vi "PH_gentec_Powermeter.Action get Info.vi"(0 "VI in":refnum<vi>, 5 "error in (no error)":errorcluster) -> (14 "VI out":refnum<vi>, 19 "error out":errorcluster)   [LabVIEW 2014, in "PH_gentec_Powermeter.lvlib"]
uses:
  PH_gentec_Powermeter.lvlib
  PH_Basics/PH_Powermeter_BaseClass/PH_Powermeter_BaseClass.State.ctl
  PH_Basics/PH_Powermeter_BaseClass/PH_Powermeter_BaseClass.lvlib
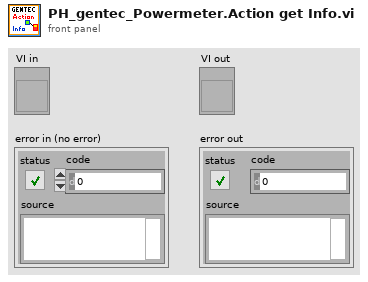
[diagram p1: front panel]
types:
  T1 = typedef "PH_Powermeter_BaseClass.lvlib/PH_Powermeter_BaseClass.State.ctl" = enum32{"off", "operating", "opened", "checked", "connected", "Sets to change", "running"}
  T2 = typedef "PH_Powermeter_BaseClass.lvlib/PH_Powermeter_BaseClass.i attribute.ctl" = cluster{"GUI References":T3, "Connection":T4, "Head Attributes":T5, "VISA resource":refnum<visa-resource-name>, "Energy":T6, "Service ID Energy":i32, "Wanted Settings":T7, "Current Settings":T7}
  T3 = typedef "PH_Powermeter_BaseClass.lvlib/PH_Powermeter_BaseClass.GUI Refs.ctl" = cluster{"Head Attributes":refnum<vi>, "Energy":refnum<vi>, "Connection":refnum<vi>, "VISA Resource":refnum<vi>, "Scaling Factor":refnum<vi>, "Range":refnum<vi>, "Wavelength":refnum<vi>, "Trigger Level":refnum<vi>, "Wanted Settings":refnum<vi>, "Current Settings":refnum<vi>}
  T4 = typedef "PH_Powermeter_BaseClass.lvlib/PH_Powermeter_BaseClass.Connection.ctl" = cluster{"failed checks":i8, "Timeout":bool, "Data read":string, "Failure":bool, "Error":bool, "State":T1}
  T5 = typedef "PH_Powermeter_BaseClass.lvlib/PH_Powermeter_BaseClass.Head Attributes.ctl" = cluster{"Instrument Type":string, "Head Version":string, "Head Name":string, "Serial Number":string, "Firmware":string, "Sensor Type":string, "MinimumRange":u32, "Maximum Range":u32, "Min Wavelength":i32, "Max Wavelength":i32}
  T6 = typedef "PH_Powermeter_BaseClass.lvlib/PH_Powermeter_BaseClass.Energy.ctl" = cluster{"current Value":dbl, "unscaled":dbl, "Scaling Factor":dbl}
  T7 = typedef "PH_Powermeter_BaseClass.lvlib/PH_gentec_BaseClass.Head Settings.ctl" = cluster{"Trigger Level":dbl, "Wavelength":u32, "Range":u32}
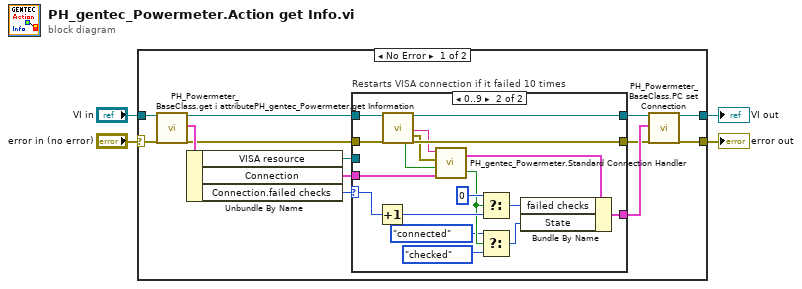
[diagram p0: block diagram]
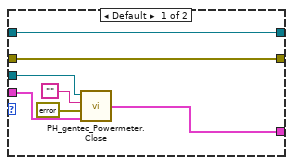
[diagram p2: hidden frame]
diagram:
  n1 = case shown="No Error" "error in (no error)" {
    selector: "error in (no error)" -> [w6 w43]
    tunnel: [w17 w43] -> w4
    tunnel: [w16 w44] -> w3
    tunnel: "VI in" -> [w7 w44]
    frame No Error {
      n2 = call "PH_Powermeter_BaseClass.get i attribute.vi"("i ref in"=w7, "error in (no error)"=w6) -> ("i ref out"=w8:refnum<vi>, "i attribute"=w11:T2, "error out"=w10:errorcluster)  [unwired: 15 in]
      n3 = Unbundle By Name(w11) -> ("VISA resource"=w5:refnum<visa-resource-name>, "Connection"=w12:T4, "Connection.failed checks"=w13:i8)
      n4 = case "Restarts VISA connection if it failed 10 times" shown="0..9" w13 {
        selector: w13 -> [_ w42]
        tunnel: w8 -> [w24 w41]
        tunnel: [w24 w40] -> w14
        tunnel: w10 -> [w23 w39]
        tunnel: [w23 w38] -> w9
        tunnel: w12 -> [w22 w37]
        tunnel: [w19 w32] -> w15
        tunnel: w5 -> [w18 _]
        frame Default {
          n5 = call "PH_gentec_Powermeter.Close.vi"("Connection in"=w22, "Device Error in"=errorcluster {"status"=FALSE, "code"=0, "source"=""} ("Device Error out"), "Error Message"="", "VISA Refnum in"=w18) -> ("Connection out"=w19:T4)
        }
        frame 0..9 {
          n6 = Increment(x=w42) -> (x+1=w30:i8)
          n7 = call "PH_gentec_Powermeter.get Information.vi"("i ref in"=w41, "error in"=w39) -> ("Timeout?"=w34:bool, "i ref out"=w40:refnum<vi>, "Error Messages"=w35:string, "Device Error out"=w36:errorcluster, "error out"=w38:errorcluster)  [unwired: 13 in]
          n8 = call "PH_gentec_Powermeter.Standard Connection Handler.vi"("Connection in"=w37, "Timeout"=w34, "Device Error"=w36, "Error"=w35) -> ("No problem"=w28:bool, "Connection out"=w33:T4)
          n9 = Select(t=i8 0, s=w28, f=w30) -> (s? t:f=w29:i8)
          n10 = Select(t=PH_Powermeter_BaseClass.State."connected" ("State"), s=w28, f=PH_Powermeter_BaseClass.State."checked") -> (s? t:f=w25:T1)
          n11 = Bundle By Name(cluster=w33, "failed checks"=w29, "State"=w25) -> (w32:T4)
        }
      }
      n12 = call "PH_Powermeter_BaseClass.PC set Connection.vi"("VI in"=w14, "Connection"=w15, "error in (no error)"=w9) -> ("VI out"=w16:refnum<vi>, "error out"=w17:errorcluster)  [unwired: 15 in]
    }
    frame Error {
    }
  }
  "error out" <- w4
  "VI out" <- w3
